vi "Init UIMessage Callbacks.vi"(8 "error in (no error)":errorcluster, 11 "Execution in":refnum<class "Execution.lvclass">) -> (0 "error out":errorcluster, 3 "Execution out":refnum<class "Execution.lvclass">)   [LabVIEW 2020, in "TSnax.lvlib" / "Execution.lvclass"]
uses:
  Execution.lvclass
  Execution.lvclass/Execution.ctl
  UIMessage Callback.vi
  Engine/Engine.lvclass
  UIMessage/UIMessage.lvclass
  C:/dev/illuminated-g/tsnax/TSnax/PropertyObject/PropertyObject.lvclass
  C:/dev/illuminated-g/tsnax/TSnax/UIMessage/UIMessage.lvclass
  C:/dev/illuminated-g/tsnax/TSnax/Execution/Execution.lvclass
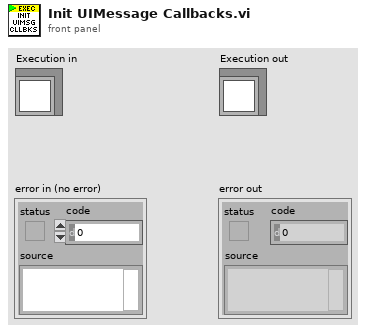
[diagram p1: front panel]
types:
  T1 = typedef "TSnax.lvlib/UIMsg.ctl" = enum16{"Unknown", "BreakOnUserRequest", "BreakOnBreakpoint", "BreakOnRunTimeError", "Trace", "TerminatingExecution", "AbortingExecution", "KillingExecutionThreads", "EndExecution", "ShutDownComplete", "StartExecution", "ProgressPercent", "ProgressText", "StartInteractiveExecution", "EndInteractiveExecution", "TerminatingInteractiveExecution", "TerminationCancelled", "ResumeFromBreak", "StartFileExecution", "EndFileExecution", "ShutDownCancelled", "LocalizationSettingChanged", "OpenWindows", "TileWindows", "CascadeWindows", "ReportChanged", "CloseWindows", "RefreshWindows", "ClientFileChanged", "DisplayReport", "ModelState_Initializing", "ModelState_Waiting", "ModelState_Identified", "ModelState_BeginTesting", "ModelState_TestingComplete", "ModelState_PostProcessingComplete", "ModelState_EnabledStateSet", "ReportLocationChanged", "GotoLocation", "PushUndoItem", "OutputMessages", "TypePaletteFileListChanged", "NonTerminatingThreadsArePreventingTermination", "ModelState_PostProcessing", "ReportCollectionChanged", "RuntimeError"}
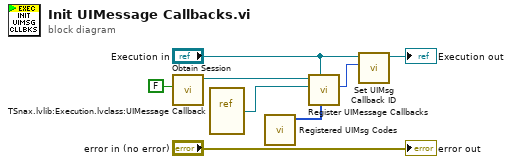
[diagram p0: block diagram]
diagram:
  n1 = call "Obtain Session.vi"("Create if needed? (T)"=FALSE) -> ("Engine out"=w6:refnum<class "Engine.lvclass">)  [unwired: 9 in, 1 out]
  n2 = vi-ref "TSnax.lvlib:Execution.lvclass:UIMessage Callback.vi"() -> (w5:refnum<vi>)
  n3 = call "Registered UIMsg Codes.vi"() -> ("UIMessage Codes"=w4:T1[])  [unwired: 11 in]
  n4 = call "Register UIMessage Callbacks.vi"("UIMessage IDs"=w4, "Owner"="Execution in", "Callback"=w5, "Engine in"=w6) -> ("Callback ID"=w2:i32)  [unwired: 5 in, 2 out]
  n5 = call "Set UIMsg Callback ID.vi"("UIMsg Callback ID"=w2, "Execution in"="Execution in") -> ("Execution out"=→"Execution out":refnum<class "Execution.lvclass">)  [unwired: 8 in, 1 out]
  "error out" <- "error in (no error)"
